vi "Averager Compute.vi"(8 "error in (no error)":errorcluster, 10 "Data":dbl[](array[numeric]), 11 "Roughness Averager in":refnum<class "Roughness Averager.lvclass">) -> (0 "error out":errorcluster, 3 "Roughness Averager out":refnum<class "Roughness Averager.lvclass">)   [LabVIEW 2018, in "Roughness Averager.lvclass"]
uses:
  Roughness Averager.lvclass
  Roughness Averager.lvclass/Roughness Averager.ctl
  Standard Averager/Standard Averager.lvclass
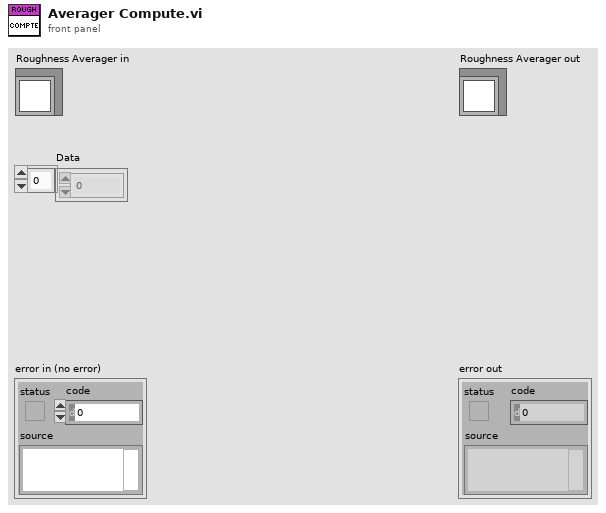
[diagram p1: front panel]
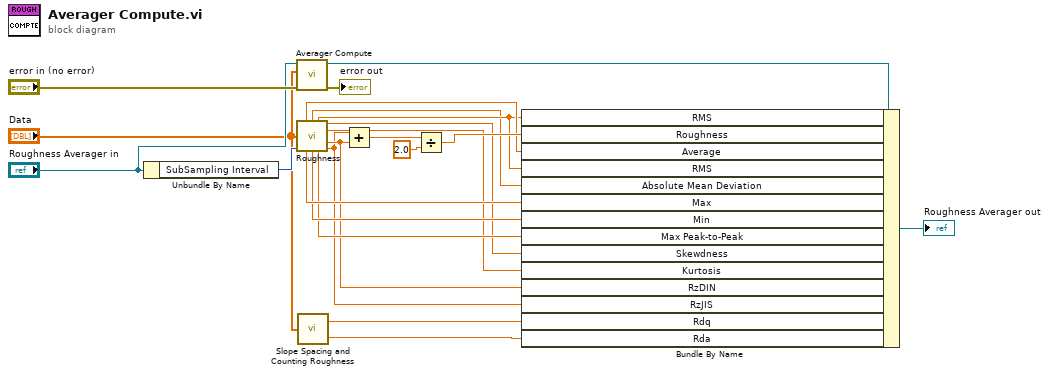
[diagram p0: block diagram]
diagram:
  n1 = Unbundle By Name("Roughness Averager in") -> ("SubSampling Interval"=w19:i32)
  n2 = call-parent "Averager Compute.vi"("error in (no error)"="error in (no error)", "Data"="Data", "Standard Averager in"="Roughness Averager in") -> ("error out"=→"error out":errorcluster, "Standard Averager out"=w15:refnum<class "Roughness Averager.lvclass">)  [unwired: 7 in]
  n3 = call "Roughness.vi"("Data"="Data", "Sub Sampling Interval (10)"=w19) -> ("Mean"=w13:dbl, "Absolute Mean Deviation"=w11:dbl, "RMS"=w12:dbl, "Skewdness"=w7:dbl, "Kurtosis"=w6:dbl, "RzDIN"=w5:dbl, "Max"=w10:dbl, "Min"=w9:dbl, "Max P-P"=w8:dbl, "RzJIS"=w4:dbl)  [unwired: 4 in]
  n4 = call "Slope Spacing and Counting Roughness.vi"("Data"="Data") -> ("Rdq"=w2:dbl, "Rda"=w1:dbl)  [unwired: 4 in]
  n5 = Add(x=w4, y=w5) -> (x+y=w18:dbl)
  n6 = Divide(x=w18, y=2.0) -> (x/y=w16:dbl)
  n7 = Bundle By Name(cluster=w15, "RMS"=w12, "Roughness"=w16, "Average"=w13, "RMS"=w12, "Absolute Mean Deviation"=w11, "Max"=w10, "Min"=w9, "Max Peak-to-Peak"=w8, "Skewdness"=w7, "Kurtosis"=w6, "RzDIN"=w5, "RzJIS"=w4, "Rdq"=w2, "Rda"=w1) -> (→"Roughness Averager out":refnum<class "Roughness Averager.lvclass">)
